vi "FeedFilterListToTree.vi"(4 "Category Names":string[](array[string]) caption="类别名称", 6 "Category Priorities":i32[](array[numeric]) caption="类别优先级", 10 "Filters":string[](array[string]) caption="过滤", 11 "Tree Ref In":refnum<vi> caption="树形控件引用输入") -> (2 "\"All\" Tag":string caption="“全部”标识符", 3 "Tree Ref Out":refnum<vi> caption="树形控件引用输出")   [LabVIEW 2016, in "NI_NPW_Filters.lvlib"]
uses:
  <resource>/dialog/NewProjectWizard/Filters/NI_NPW_Filters.lvlib
panel:
  in  "\"All\"":string="全部" caption="“全部”"
  in  "Test Tree":string(tree) caption="测试目录树"
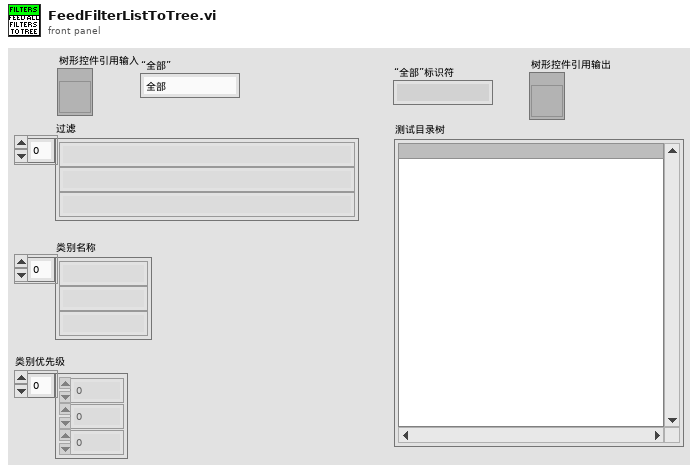
[diagram p1: front panel]
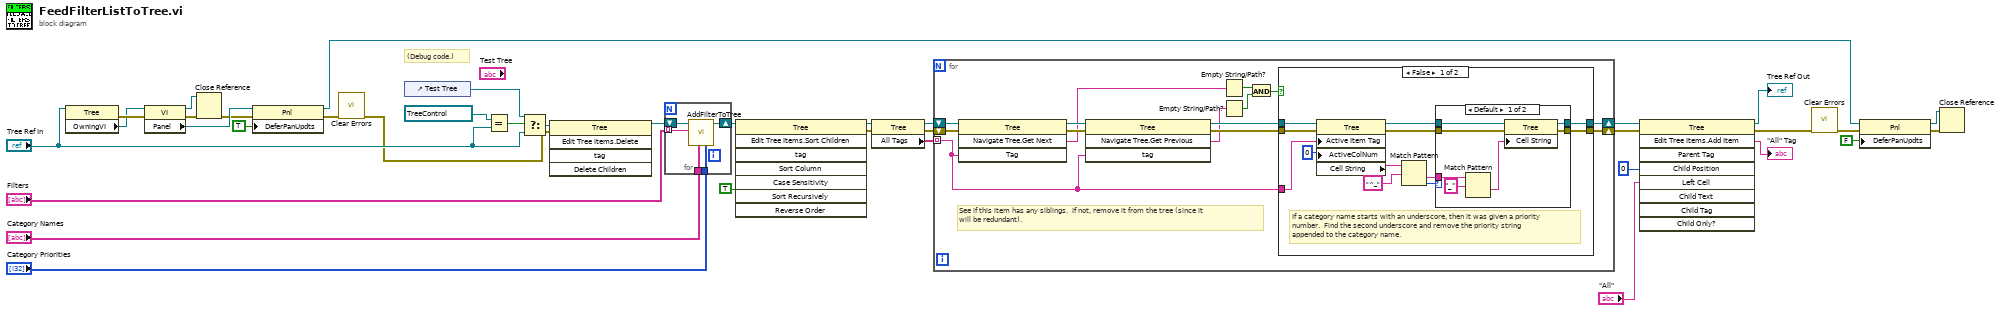
[diagram p0: block diagram]
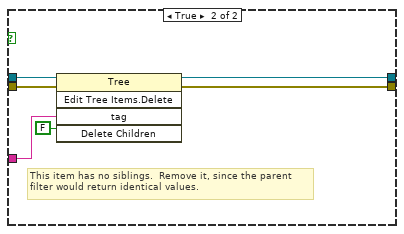
[diagram p3: hidden frame]
diagram:
  # "(Debug code.)"
  n1 = property class="Tree"(reference="Tree Ref In") -> (error out=w17:errorcluster, "OwningVI"=w16:refnum<vi>)  [unwired: 1 in, 1 out]
  n2 = property class="VI"(reference=w16, error in=w17) -> (reference out=w3:refnum<vi>, error out=w15:errorcluster, "Panel"=w14:refnum<vi>)
  n3 = Close Reference(reference=w3, error in (no error)=w15) -> (error out=w4:errorcluster)
  n4 = property class="Pnl"(reference=w14, error in=w4, "DeferPanUpdts"=TRUE ("Defer Panel Updates")) -> (reference out=w7:refnum<vi>, error out=w12:errorcluster)
  n5 = call <vilib>:"Clear Errors.vi"("error in (no error)"=w12) -> ("error out"=w11:errorcluster)  [unwired: 5 in, 1 out]
  n6 = control-ref of="Test Tree"() -> (w35:refnum<vi>)
  n7 = Equal?(x=refnum<vi> refnum ("Tree Refnum"), y="Tree Ref In") -> (x = y?=w37:bool)
  n8 = Select(t=w35, s=w37, f="Tree Ref In") -> (s? t:f=w25:refnum<vi>)
  n9 = invoke class="Tree" method="Edit Tree Items.Delete"(reference=w25, error in=w11) -> (reference out=w26:refnum<vi>)  [unwired: 3 in, 4 out]
  n10 = for {
    tunnel: "Filters" -> [w41] mode=indexing
    shift-right: [w40] -> w33
    shift-left: w26 -> [w42]
    tunnel: "Category Names" -> [w39]
    tunnel: "Category Priorities" -> [w38]
    n11 = call <resource>:"AddFilterToTree.vi"("Category Priorities"=w38, "Category Names"=w39, "Filter"=w41, "Tree Refnum In"=w42) -> ("Tree Refnum Out"=w40:refnum<vi>)  [unwired: 7 in]
  }
  n12 = invoke class="Tree" method="Edit Tree Items.Sort Children"(reference=w33, "Sort Recursively"=TRUE ("Sort Recursively?")) -> (reference out=w24:refnum<vi>, error out=w31:errorcluster)  [unwired: 6 in, 6 out]
  n13 = property class="Tree"(reference=w24, error in=w31) -> (reference out=w22:refnum<vi>, error out=w23:errorcluster, "All Tags"=w21:string[])
  n14 = for {
    shift-right: [w55] -> w19
    shift-left: w23 -> [w56]
    tunnel: w21 -> [w48] mode=indexing
    shift-right: [w54] -> w20
    shift-left: w22 -> [w52]
    # "See if this item has any siblings.  If not, remove it from the tree (since it\nwill be redundant)."
    n15 = invoke class="Tree" method="Navigate Tree.Get Next"(reference=w52, error in=w56, "Tag"=w48) -> (reference out=w50:refnum<vi>, error out=w53:errorcluster, "Navigate Tree:Get Next Item"=w47:string)  [unwired: 1 in, 1 out]
    n16 = invoke class="Tree" method="Navigate Tree.Get Previous"(reference=w50, error in=w53, "tag"=w48) -> (reference out=w49:refnum<vi>, error out=w51:errorcluster, "Navigate Tree:Get Previous"=w46:string)  [unwired: 1 in, 1 out]
    n17 = Empty String/Path?(string/path=w47) -> (empty?=w45:bool)
    n18 = Empty String/Path?(string/path=w46) -> (empty?=w44:bool)
    n19 = And(x=w45, y=w44) -> (x .and. y?=w43:bool)
    n20 = case shown="False" w43 {
      tunnel: [w62 w79] -> w55
      tunnel: [w60 w78] -> w54
      tunnel: w51 -> [w59 w82]
      tunnel: w49 -> [w58 w83]
      tunnel: w48 -> [w57 w81]
      frame False {
        # "If a category name starts with an underscore, then it was given a priority number.  Find the second underscore and remove the priority string appended to the category name."
        n21 = property class="Tree"(reference=w58, error in=w59, "Active Item Tag"=w57, "ActiveColNum"=0 ("Active Cell:Active Column Number")) -> (reference out=w63:refnum<vi>, error out=w64:errorcluster, "Cell String"=w67:string)
        n22 = Match Pattern(string=w67, regular expression="^_") -> (after substring=w61:string, offset past match=w65:i32)  [unwired: 1 in, 2 out]
        n23 = case shown="Default" w65 {
          tunnel: w64 -> [w72 w77]
          tunnel: w63 -> [w73 w76]
          tunnel: [w70 w77] -> w62
          tunnel: [w69 w76] -> w60
          tunnel: w61 -> [w75 _]
          frame Default {
            n24 = Match Pattern(string=w75, regular expression="_") -> (after substring=w71:string)  [unwired: 1 in, 3 out]
            n25 = property class="Tree"(reference=w73, error in=w72, "Cell String"=w71) -> (reference out=w69:refnum<vi>, error out=w70:errorcluster)
          }
          frame -1 {
          }
        }
      }
      frame True {
        # "This item has no siblings.  Remove it, since the parent\nfilter would return identical values."
        n26 = invoke class="Tree" method="Edit Tree Items.Delete"(reference=w83, error in=w82, "tag"=w81, "Delete Children"=FALSE ("Delete Children?")) -> (reference out=w78:refnum<vi>, error out=w79:errorcluster)  [unwired: 1 in, 3 out]
      }
    }
  }
  n27 = invoke class="Tree" method="Edit Tree Items.Add Item"(reference=w20, error in=w19, "Child Position"=0, "Left Cell"="\"All\"") -> (reference out=→"Tree Ref Out":refnum<vi>, error out=w10:errorcluster, "Edit Tree Items:Add Item"=→"\"All\" Tag":string)  [unwired: 5 in, 6 out]
  n28 = call <vilib>:"Clear Errors.vi"("error in (no error)"=w10) -> ("error out"=w9:errorcluster)  [unwired: 5 in, 1 out]
  n29 = property class="Pnl"(reference=w7, error in=w9, "DeferPanUpdts"=FALSE ("Defer Panel Updates")) -> (reference out=w5:refnum<vi>, error out=w6:errorcluster)
  n30 = Close Reference(reference=w5, error in (no error)=w6) -> ()  [unwired: 1 out]
